vi "Teleop Climb V.5.0.vi"   [LabVIEW 2016]
uses:
  Robot Global Data V.5.0.vi
types:
  T1 = typedef "WPI_MotorControlDeviceRef.ctl" = cluster{"DeviceStatus":errorcluster, "Type":T2, "PWM":cluster{"PWM Channel":T3, "DeadBand":T4}, "CAN":cluster{"Device Number":u8, "SetOutput VI Ref":variant, "GetOutput VI Ref":variant, "Enable VI Ref":variant, "Disable VI Ref":variant, "Data":variant}, "Invert":bool}
  T2 = typedef "WPI_MotorControlType.ctl" = enum16{"PWM", "CAN"}
  T3 = typedef "FPGA_DIOPWMChannel.ctl" = enum8{"PWM 0", "PWM 1", "PWM 2", "PWM 3", "PWM 4", "PWM 5", "PWM 6", "PWM 7", "PWM 8", "PWM 9", "PWM MXP 0", "PWM MXP 1", "PWM MXP 2", "PWM MXP 3", "PWM MXP 4", "PWM MXP 5", "PWM MXP 6", "PWM MXP 7", "PWM MXP 8", "PWM MXP 9", "Invalid"}
  T4 = typedef "WPI_PWMDeadband.ctl" = cluster{"Name":string, "maxPositivePwm":i32, "minPositivePwm":i32, "centerPwm":i32, "maxNegativePwm":i32, "minNegativePwm":i32, "angularRange":u16}
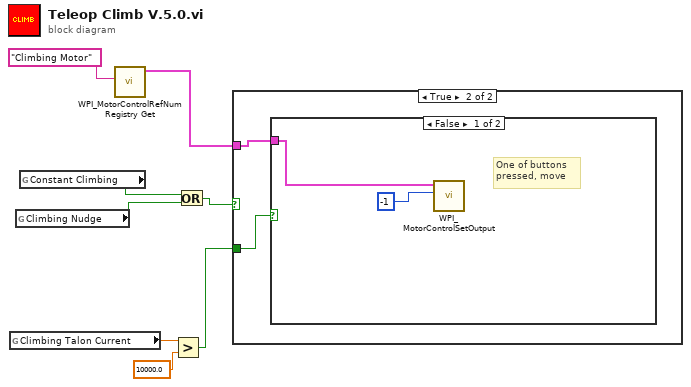
[diagram p0: block diagram]
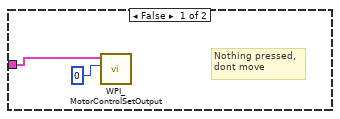
[diagram p2: hidden frame]
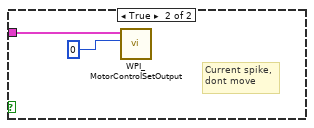
[diagram p3: hidden frame]
diagram:
  n1 = global read "Robot Global Data V.5.0.vi" "Climbing Talon Current"() -> (w3:dbl)
  n2 = global read "Robot Global Data V.5.0.vi" "Climbing Nudge"() -> (w4:bool)
  n3 = global read "Robot Global Data V.5.0.vi" "Constant Climbing"() -> (w5:bool)
  n4 = call <vilib>:"WPI_MotorControlRefNum Registry Get.vi"("refnum name"="Climbing Motor") -> ("MotorControlDevRef"=w7:T1)  [unwired: 9 in, 1 out]
  n5 = Greater?(x=w3, y=10000.0) -> (0:w1:bool)
  n6 = Or(x=w5, y=w4) -> (x .or. y?=w6:bool)
  n7 = case shown="True" w6 {
    tunnel: w7 -> [w10 w12]
    tunnel: w1 -> [_ w11]
    frame False {
      # "Nothing pressed,\ndont move"
      n8 = call <vilib>:"WPI_MotorControlSetOutput.vi"("Output"=0, "MotorControlDevRef"=w10) -> ()  [unwired: 7 in, 3 out]
    }
    frame True {
      n9 = case shown="False" w11 {
        tunnel: w12 -> [w13 w16]
        frame False {
          # "One of buttons \npressed, move"
          n10 = call <vilib>:"WPI_MotorControlSetOutput.vi"("Output"=-1, "MotorControlDevRef"=w13) -> ()  [unwired: 7 in, 3 out]
        }
        frame True {
          # "Current spike,\ndont move"
          n11 = call <vilib>:"WPI_MotorControlSetOutput.vi"("Output"=0, "MotorControlDevRef"=w16) -> ()  [unwired: 7 in, 3 out]
        }
      }
    }
  }
